vi "AllowEdgeStartCheck.vi"(0 "reference in":refnum<class "SequenceDiagramGraph.lvclass">, 1 "EdgeStartNode":refnum<class "AbstractNode.lvclass">, 2 "GraphButton":u32, 5 "error in (no error)":errorcluster) -> (14 "reference out":refnum<class "SequenceDiagramGraph.lvclass">, 16 "Allowed":bool, 19 "error out":errorcluster)   [LabVIEW 2014, in "SequenceDiagramGraph.lvclass"]
uses:
  <resource>/Framework/Providers/Open_GDS/UML/SequenceDiagramGraph_class/SequenceDiagramGraph.lvclass
  <resource>/Framework/Providers/Open_GDS/UML/AbstractNode_class/AbstractNode.lvclass
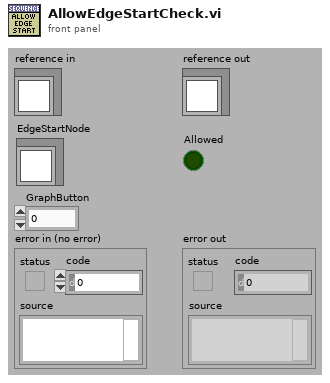
[diagram p1: front panel]
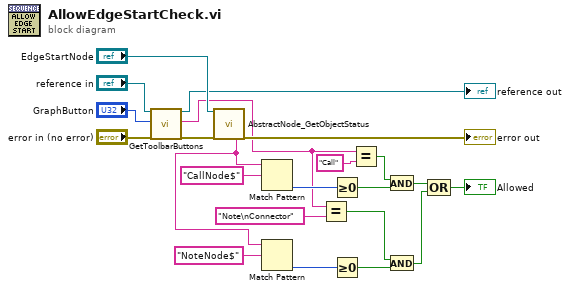
[diagram p0: block diagram]
diagram:
  n1 = call-dynamic "GetToolbarButtons.vi"("reference in"="reference in", "GraphButton"="GraphButton", "error in (no error)"="error in (no error)") -> ("reference out"=→"reference out":refnum<class "SequenceDiagramGraph.lvclass">, "Text"=w3:string, "error out"=w16:errorcluster)  [unwired: 12 in, 2 out]
  n2 = call <resource>:"AbstractNode_GetObjectStatus.vi"("reference in"="EdgeStartNode", "error in (no error)"=w16) -> ("Class name"=w5:string, "error out"=→"error out":errorcluster)  [unwired: 16 out]
  n3 = Match Pattern(string=w5, regular expression="CallNode$") -> (offset past match=w8:i32)  [unwired: 4 out]
  n4 = Match Pattern(string=w5, regular expression="NoteNode$") -> (offset past match=w14:i32)  [unwired: 4 out]
  n5 = Equal?(x=w3, y="Note\nConnector" ("Text")) -> (x = y?=w13:bool)
  n6 = Greater Or Equal To 0?(x=w8) -> (x >= 0?=w10:bool)
  n7 = Greater Or Equal To 0?(x=w14) -> (x >= 0?=w12:bool)
  n8 = Equal?(x=w3, y="Call" ("Text")) -> (x = y?=w9:bool)
  n9 = And(x=w9, y=w10) -> (x .and. y?=w6:bool)
  n10 = And(x=w13, y=w12) -> (x .and. y?=w11:bool)
  n11 = Compound Arithmetic op=OR(w6, w11) -> (→"Allowed":bool)
